vi "read_layer.vi"(10 "IMAGE PATH":path=path "C:/Users/swift/Desktop/Python/imec/Data/SKFX.300x300.Binning.2.frame.1.Gain.1.time.5.HDR-V3_corrected.hdr", 11 "Band":i32) -> (1 "Layer":sgl[][](array[numeric]), 3 "Image":u8[][](array[numeric]))   [LabVIEW 2018]
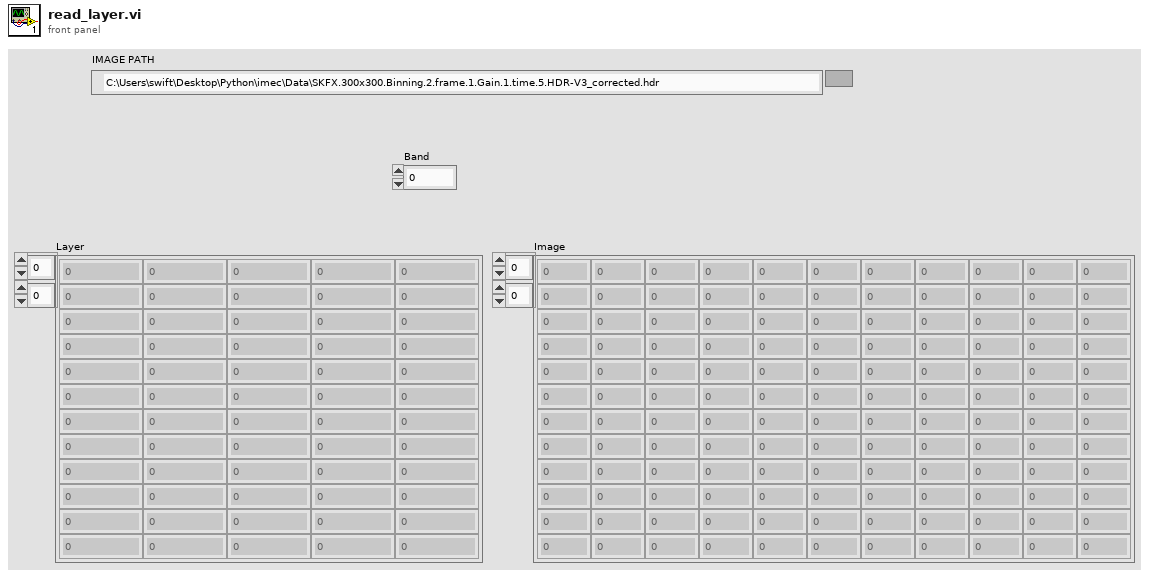
[diagram p1: front panel]
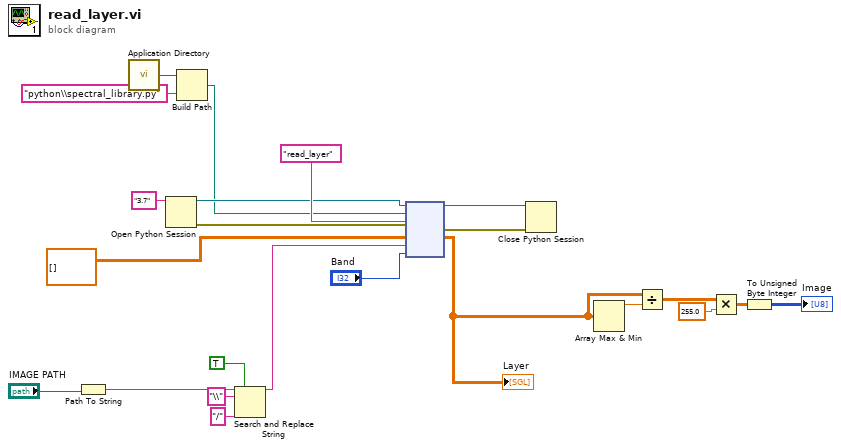
[diagram p0: block diagram]
diagram:
  n1 = Path To String(path="IMAGE PATH") -> (string=w20:string)
  n2 = call <vilib>:"Application Directory.vi"() -> ("Application Directory"=w12:path)
  n3 = Open Python Session(python version="3.7" ("version Python")) -> (session out=w10:refnum<k35>, error out=w22:errorcluster)  [unwired: 2 in]
  n4 = Build Path(base path=w12, name or relative path="python\\spectral_library.py" ("nom ou chemin relatif")) -> (appended path=w9:path)
  n5 = Search and Replace String(replace all?=TRUE ("replace all? (F)"), input string=w20, search string="\\", replace string="/" ("replace string (\"\")")) -> (result string=w15:string)  [unwired: 4 in, 3 out]
  n6 = node(w10, w9, "read_layer" ("nom de la fonction"), w22, sgl[][] [], w15, "Band") -> (w14:refnum<k35>, w13:errorcluster, w2:sgl[][])  [unwired: 2 in, 2 out]
  "Layer" <- w2
  n7 = Close Python Session(session in=w14, error in=w13) -> ()  [unwired: 1 out]
  n8 = Array Max & Min(array=w2) -> (max value=w6:sgl)  [unwired: 3 out]
  n9 = Divide(x=w2, y=w6) -> (x/y=w4:sgl[][])
  n10 = Multiply(x=w4, y=sgl 255.0) -> (x*y=w3:sgl[][])
  n11 = To Unsigned Byte Integer(number=w3) -> (unsigned 8bit integer=→"Image":u8[][])
